vi "QueryWavelength.vi"(8 "error in (no error)":errorcluster, 11 "HRS_Spectrometer in":refnum<class "HRS_Spectrometer.lvclass">) -> (0 "error out":errorcluster, 3 "HRS_Spectrometer out":refnum<class "HRS_Spectrometer.lvclass">)   [LabVIEW 2023, in "HRS_Spectrometer.lvlib" / "HRS_Spectrometer.lvclass"]
uses:
  HRS_Spectrometer.lvclass
  HRS_Spectrometer.lvclass/HRS_Spectrometer.ctl
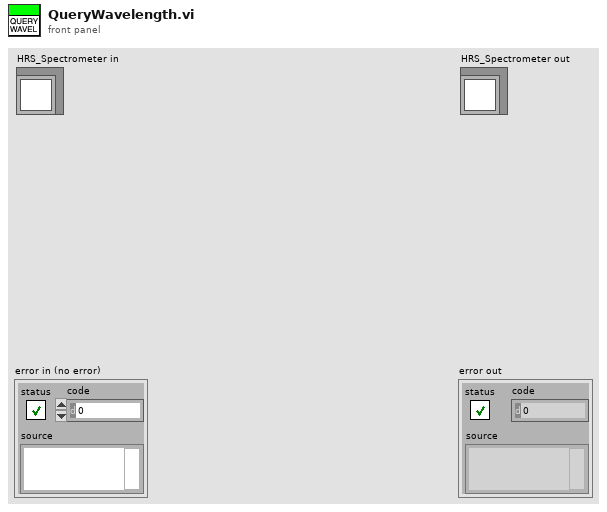
[diagram p1: front panel]
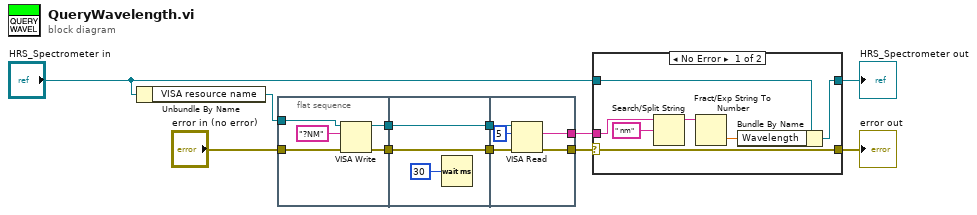
[diagram p0: block diagram]
diagram:
  n1 = Unbundle By Name("HRS_Spectrometer in") -> ("VISA resource name"=w7:refnum<visa-resource-name>)
  n2 = flat-sequence {
    tunnel: [w15] -> w11
    tunnel: [w14] -> w10
    tunnel: w7 -> [w13]
    tunnel: "error in (no error)" -> [w12]
    tunnel: w11 -> [w19]
    tunnel: w10 -> [w18]
    tunnel: [w19] -> w9
    tunnel: [w18] -> w8
    tunnel: w9 -> [w23]
    tunnel: w8 -> [w24]
    tunnel: [w22] -> w5
    tunnel: [w21] -> w4
    frame #0 {
      n3 = VISA Write(VISA resource name=w13, write buffer="?NM", error in (no error)=w12) -> (VISA resource name out=w15:refnum<visa-resource-name>, error out=w14:errorcluster)  [unwired: 1 out]
    }
    frame #1 {
      n4 = Wait (ms)(milliseconds to wait=u32 30) -> ()  [unwired: 1 out]
    }
    frame #2 {
      n5 = VISA Read(VISA resource name=w23, byte count=u32 5, error in (no error)=w24) -> (read buffer=w22:string, error out=w21:errorcluster)  [unwired: 2 out]
    }
  }
  n6 = case shown="No Error" w4 {
    selector: w4 -> [w26 w33]
    tunnel: w5 -> [w31 _]
    tunnel: [w28 w32] -> w2
    tunnel: [w26 w33] -> w3
    tunnel: "HRS_Spectrometer in" -> [w25 w32]
    frame No Error {
      n7 = Search/Split String(string=w31, search string/char (-)=" nm") -> (substring before match=w29:string)  [unwired: 1 in, 2 out]
      n8 = Fract/Exp String To Number(string=w29) -> (number=w27:dbl)  [unwired: 3 in, 1 out]
      n9 = Bundle By Name(cluster=w25, "Wavelength"=w27) -> (w28:refnum<class "HRS_Spectrometer.lvclass">)
    }
    frame Error {
    }
  }
  "error out" <- w3
  "HRS_Spectrometer out" <- w2
